vi "GETCCD.vi"(1 "lines":u32, 2 "pixel":u32=600, 3 "zadr":u32=1, 4 "lfkt":i32=1) -> (0 "Data Values":u32[](graph))   [LabVIEW 2014]
uses:
  ESLSCDLL.dll
panel:
  # "lines for  FFTs, or 0 else"
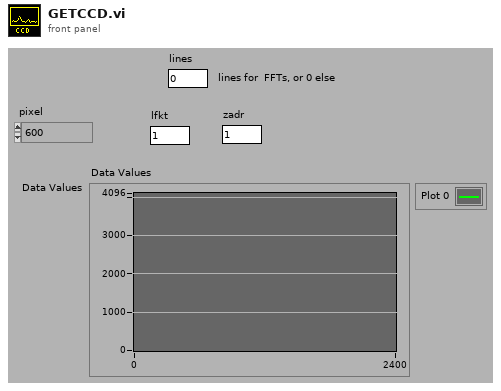
[diagram p1: front panel]
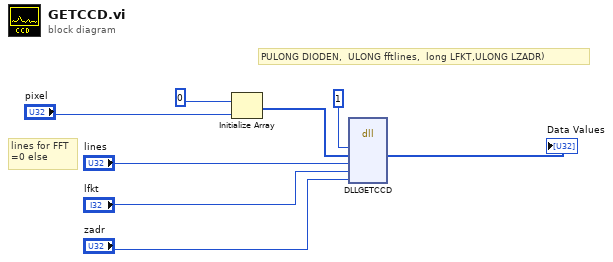
[diagram p0: block diagram]
diagram:
  # "lines for FFT\n=0 else"
  # "PULONG DIODEN, \tULONG fftlines,  long LFKT,ULONG LZADR)"
  n1 = Initialize Array(u32 0, "pixel") -> (w3:u32[])
  n2 = dll-call lib="C:/Users/Gerhard/Documents/New64/lv/1cam/board.vis/ESLSCDLL.dll" fn="DLLGETCCD"("drv"=u32 1, "dioden"=w3, "fftlines"="lines", "fkt"="lfkt", "zadr"="zadr") -> ("dioden"=→"Data Values":u32[])  [unwired: 8 in, 2 out]
